vi "InitFT.vi"(3 "Timing parameters":T1={"Sample Rate"=1000.0, "Samples to Read"=100}, 5 "Channel Parameters":T2={"Maximum Value"=10.0, "Minimum Value"=-10.0, "Channel"=""}) -> (0 "error out":errorcluster, 1 "task out":refnum<k21>)   [LabVIEW 2012]
uses:
  <vilib>/DAQmx/create/channels.llb/DAQmx Create Channel (AI-Voltage-Basic).vi
  <vilib>/DAQmx/configure/timing.llb/DAQmx Timing (Sample Clock).vi
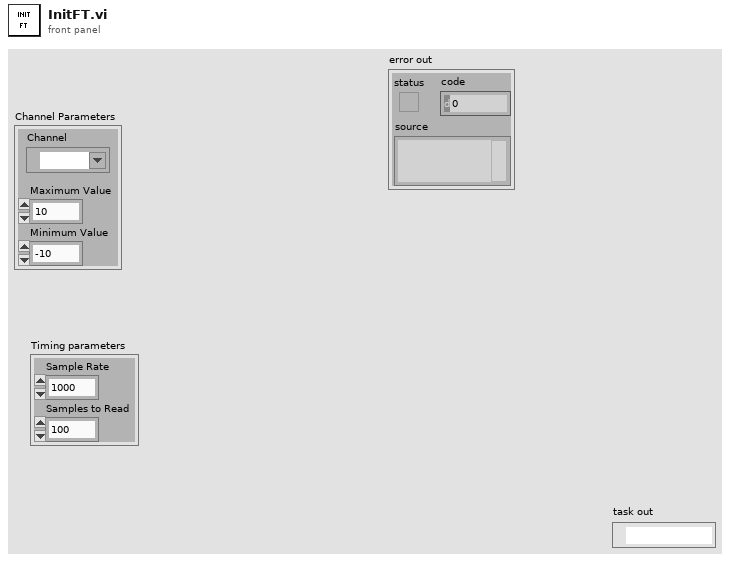
[diagram p1: front panel]
types:
  T1 = cluster{"Sample Rate":dbl, "Samples to Read":i32}
  T2 = cluster{"Maximum Value":dbl, "Minimum Value":dbl, "Channel":tag}
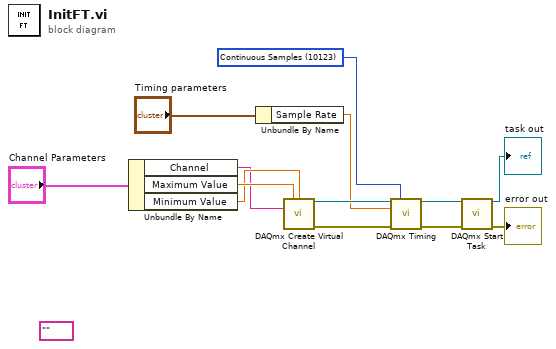
[diagram p0: block diagram]
diagram:
  (unwired) tag "" ("Channel")
  w11 = 10123 items=["Finite Samples"=10178, "Continuous Samples"=10123] ("sample mode")
  n1 = Unbundle By Name("Channel Parameters") -> ("Channel"=w1:tag, "Maximum Value"=w7:dbl, "Minimum Value"=w6:dbl)
  n2 = Unbundle By Name("Timing parameters") -> ("Sample Rate"=w5:dbl)
  n3 = call-poly <vilib>:"DAQmx Create Virtual Channel.vi"("maximum value"=w7, "minimum value"=w6, "physical channels"=w1) -> ("task out"=w12:refnum<k21>, "error out"=w13:errorcluster)  [unwired: 11 in]
  n4 = call-poly <vilib>:"DAQmx Timing.vi"("task/channels in"=w12, "sample mode"=w11, "rate"=w5, "error in"=w13) -> ("task out"=w10:refnum<k21>, "error out"=w9:errorcluster)  [unwired: 10 in]
  n5 = call <vilib>:"DAQmx Start Task.vi"("task/channels in"=w10, "error in"=w9) -> ("task out"=→"task out":refnum<k21>, "error out"=→"error out":errorcluster)  [unwired: 12 in]
